vi "BooleanSchmittTrigger.vi"(7 "Upper limit":dbl, 8 "error in (no error)":errorcluster, 9 "Lower limit":dbl, 10 "Current Value":dbl, 11 "Utilities in":refnum<class "Utilities.lvclass">) -> (0 "error out":errorcluster, 2 "Scmitt result":bool, 3 "Utilities out":refnum<class "Utilities.lvclass">)   [LabVIEW 2018, in "Utilities.lvclass"]
uses:
  Utilities.lvclass
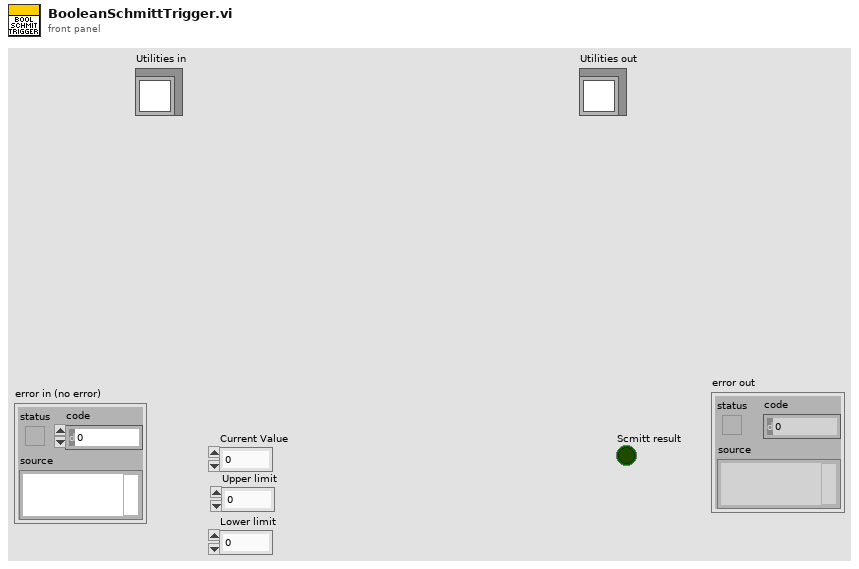
[diagram p1: front panel]
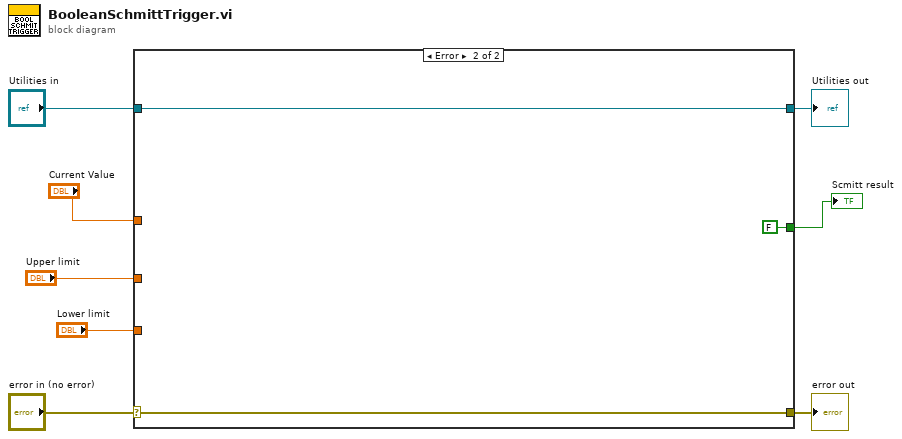
[diagram p0: block diagram]
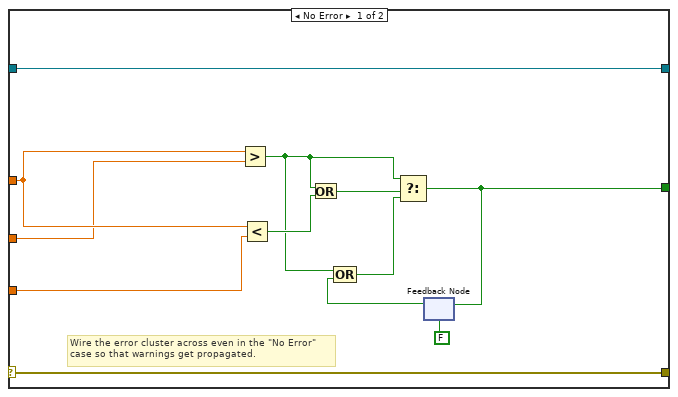
[diagram p2: hidden frame]
diagram:
  n1 = case shown="Error" "error in (no error)" {
    selector: "error in (no error)" -> [w19 w23]
    tunnel: [w19 w23] -> w7
    tunnel: [w20 w22] -> w5
    tunnel: "Utilities in" -> [w20 w22]
    tunnel: [w12 FALSE] -> w4
    tunnel: "Current Value" -> [w11 _]
    tunnel: "Upper limit" -> [w10 _]
    tunnel: "Lower limit" -> [w9 _]
    frame No Error {
      # "Wire the error cluster across even in the \"No Error\"\ncase so that warnings get propagated."
      n2 = Greater?(x=w11, y=w10) -> (0:w16:bool)
      n3 = Less?(x=w11, y=w9) -> (x < y?=w18:bool)
      n4 = Or(x=w16, y=w18) -> (x .or. y?=w17:bool)
      n5 = feedback #1(FALSE) -> (w14:bool)
      n6 = Compound Arithmetic op=OR(w16, w14) -> (w15:bool)
      n7 = Select(t=w16, s=w17, f=w15) -> (s? t:f=w12:bool)
      n8 = feedback-in #1(w12) -> ()
    }
    frame Error {
    }
  }
  "error out" <- w7
  "Utilities out" <- w5
  "Scmitt result" <- w4
